vi "Command_write.vi"(8 "错误输入（无错误）":errorcluster, 9 "Status code":string, 10 "Data":string, 11 "VISA引用句柄输入":refnum<visa-resource-name>) -> (0 "错误输出":errorcluster, 2 "return count":u32, 3 "VISA引用句柄输出":refnum<visa-resource-name>)   [LabVIEW 2014]
panel:
  out "字符串":string
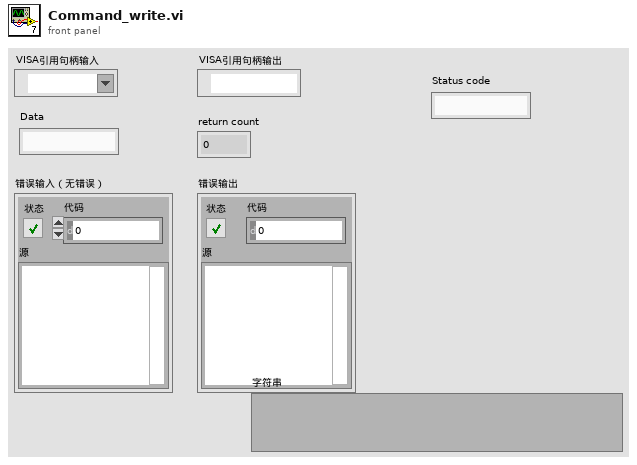
[diagram p1: front panel]
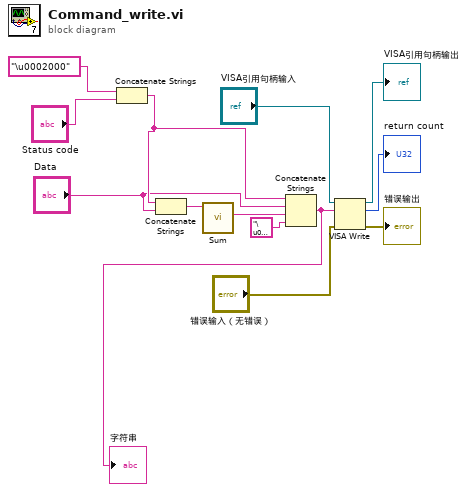
[diagram p0: block diagram]
diagram:
  n1 = Concatenate Strings("\u0002000", "Status code") -> (w4:string)
  n2 = Concatenate Strings(w4, "Data") -> (w13:string)
  n3 = call "Sum.vi"("连接的字符串"=w13) -> ("string"=w12:string)  [unwired: 8 in, 2 out]
  n4 = Concatenate Strings(w4, "Data", w12, "\u0003") -> (w5:string)
  "字符串" <- w5
  n5 = VISA Write(VISA resource name="VISA引用句柄输入", write buffer=w5, error in (no error)="错误输入（无错误）") -> (VISA resource name out=→"VISA引用句柄输出":refnum<visa-resource-name>, return count=→"return count":u32, error out=→"错误输出":errorcluster)
